vi "Handle Trace.vi"(8 "error in (no error)":errorcluster, 10 "Sequence Context":refnum<k7>, 11 "SequenceViewPanel in":refnum<class "SequenceViewPanel.lvclass">) -> (0 "error out":errorcluster, 3 "SequenceViewPanel out":refnum<class "SequenceViewPanel.lvclass">)   [LabVIEW 2020, in "TSnax UI.lvlib" / "SequenceViewPanel.lvclass"]
uses:
  SequenceViewPanel.lvclass
  Trace Marker.ctl
  TSnax/SequenceFile/SequenceFile.lvclass
  SequenceViewPanel.lvclass/SequenceViewPanel.ctl
  TSnax/Engine/Engine.lvclass
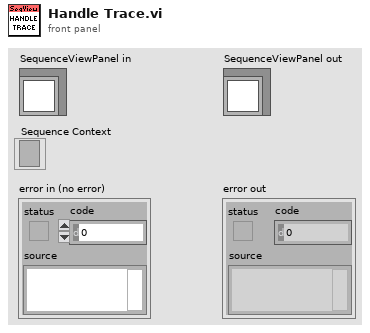
[diagram p1: front panel]
types:
  T1 = typedef "TSnax UI.lvlib/SequenceViewPanel.lvclass/Trace Marker.ctl" = cluster{"TSnax:SequenceFile":refnum<class "SequenceFile.lvclass">, "SequenceIndex":i32, "StepGroup":i32, "PreviousStepIndex":i32, "NextStepIndex":i32}
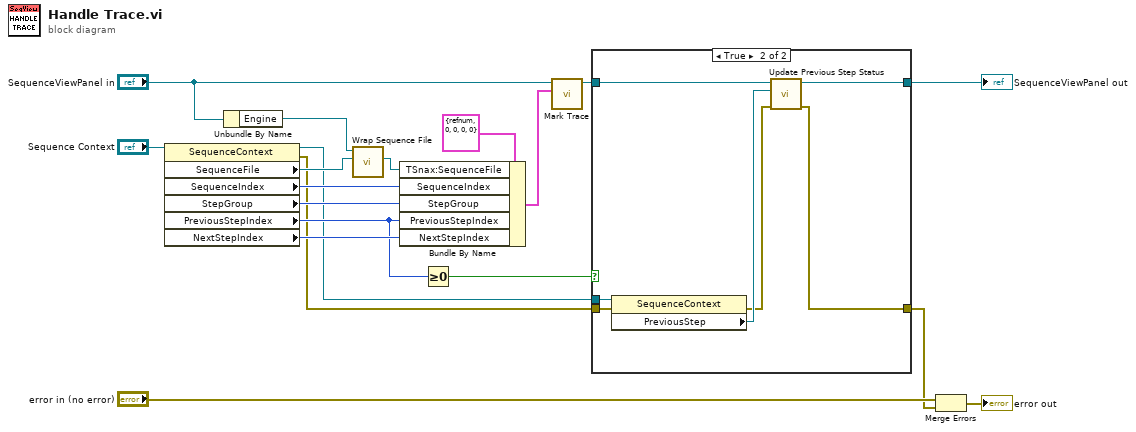
[diagram p0: block diagram]
diagram:
  n1 = property class="SequenceContext"(reference="Sequence Context") -> (reference out=w3:refnum<k7>, error out=w2:errorcluster, "SequenceFile"=w13:refnum<k7>, "SequenceIndex"=w16:i32, "StepGroup"=w15:i32, "PreviousStepIndex"=w7:i32, "NextStepIndex"=w9:i32)  [unwired: 1 in]
  n2 = Unbundle By Name("SequenceViewPanel in") -> ("Engine"=w12:refnum<class "Engine.lvclass">)
  n3 = call "Wrap Sequence File.vi"("TS SequenceFile"=w13, "Engine in"=w12) -> ("TSnax:SequenceFile"=w11:refnum<class "SequenceFile.lvclass">)  [unwired: 7 in, 2 out]
  n4 = Bundle By Name(cluster=T1 {"TSnax:SequenceFile"=refnum, "SequenceIndex"=0, "StepGroup"=0, "PreviousStepIndex"=0, "NextStepIndex"=0} ("Trace Marker"), "TSnax:SequenceFile"=w11, "SequenceIndex"=w16, "StepGroup"=w15, "PreviousStepIndex"=w7, "NextStepIndex"=w9) -> (w8:T1)
  n5 = Greater Or Equal To 0?(x=w7) -> (x >= 0?=w6:bool)
  n6 = call "Mark Trace.vi"("Trace Marker"=w8, "SequenceViewPanel in"="SequenceViewPanel in") -> ("SequenceViewPanel out"=w5:refnum<class "SequenceViewPanel.lvclass">)  [unwired: 8 in, 1 out]
  n7 = case shown="True" w6 {
    tunnel: w5 -> [w21 w28]
    tunnel: [w21 w27] -> w4
    tunnel: w3 -> [_ w26]
    tunnel: w2 -> [w20 w25]
    tunnel: [w20 w22] -> w1
    frame False {
    }
    frame True {
      n8 = property class="SequenceContext"(reference=w26, error in=w25) -> (error out=w23:errorcluster, "PreviousStep"=w24:refnum<k7>)  [unwired: 1 out]
      n9 = call "Update Previous Step Status.vi"("error in (no error)"=w23, "PreviousStep"=w24, "SequenceViewPanel in"=w28) -> ("error out"=w22:errorcluster, "SequenceViewPanel out"=w27:refnum<class "SequenceViewPanel.lvclass">)  [unwired: 7 in]
    }
  }
  "SequenceViewPanel out" <- w4
  n10 = Merge Errors("error in (no error)", w1) -> (→"error out":errorcluster)
